vi "OperateControlPosition.vi"   [LabVIEW 2011]
uses:
  <vilib>/Utility/miscctls.llb/LVPositionTypeDef.ctl
types:
  T1 = typedef "LVPositionTypeDef.ctl" = cluster{"Left":i32, "Top":i32}
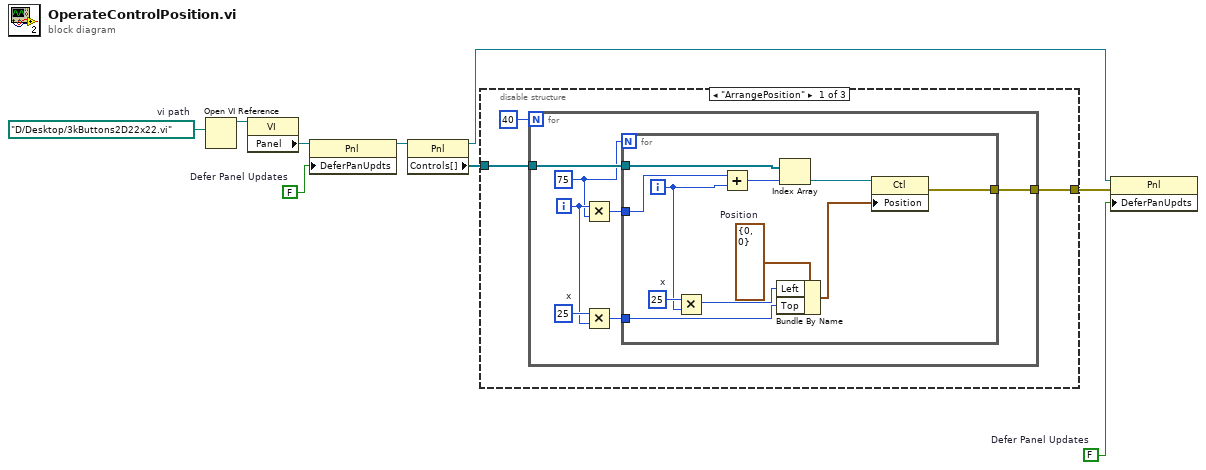
[diagram p0: block diagram]
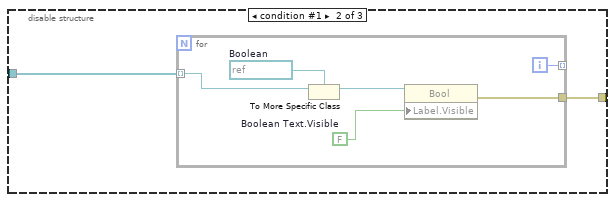
[diagram p2: hidden frame]
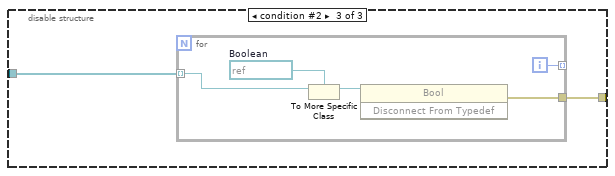
[diagram p3: hidden frame]
diagram:
  w3 = FALSE  # Defer Panel Updates
  w5 = FALSE  # Defer Panel Updates
  w7 = path "D:/Desktop/3kButtons2D22x22.vi"  # vi path
  n1 = Open VI Reference(vi path=w7) -> (vi reference=w8:refnum<vi>)  [unwired: 5 in, 1 out]
  n2 = property class="VI"(reference=w8) -> ("Panel"=w6:refnum<vi>)  [unwired: 1 in, 2 out]
  n3 = property class="Pnl"(reference=w6, "DeferPanUpdts"=w5) -> (reference out=w1:refnum<vi>)  [unwired: 1 in, 1 out]
  n4 = property class="Pnl"(reference=w1) -> (reference out=w2:refnum<vi>, "Controls[]"=w9:refnum<vi>[])  [unwired: 1 in, 1 out]
  n5 = disable-structure shown="\"ArrangePosition\"" {
    disable-tunnel: w9 -> [w12 w32 w40]
    disable-tunnel: [w11 w31 w39] -> w4
    frame condition #0 (active) {
      n6 = for {
        N: 40 -> [_]
        tunnel: w12 -> [w19]
        tunnel: [w18] -> w11
        i -> [w15]
        w17 = 25  # x
        w13 = 75
        n7 = Multiply(x=w15, y=w13) -> (x*y=w14:i32)
        n8 = Multiply(x=w17, y=w15) -> (x*y=w16:i32)
        n9 = for {
          N: w13 -> [_]
          tunnel: w19 -> [w30]
          tunnel: [w29] -> w18
          tunnel: w16 -> [w24]
          tunnel: w14 -> [w21]
          i -> [w20]
          w26 = 25  # x
          w28 = T1 {"Left"=0, "Top"=0}  # Position
          n10 = Multiply(x=w26, y=w20) -> (x*y=w25:i32)
          n11 = Add(x=w21, y=w20) -> (x+y=w22:i32)
          n12 = Bundle By Name(cluster=w28, "Left"=w25, "Top"=w24) -> (w27:T1)
          n13 = Index Array(array=w30, index=w22) -> (element=w23:refnum<vi>)
          n14 = property class="Ctl"(reference=w23, "Position"=w27) -> (error out=w29:errorcluster)  [unwired: 1 in, 1 out]
        }
      }
    }
    frame condition #1 {
      n15 = for {
        tunnel: w32 -> [w37] mode=indexing
        tunnel: [w38] -> w31
        tunnel: [w34] -> _ mode=indexing
        i -> [w34]
        w33 = FALSE  # Boolean Text.Visible
        w35 = refnum<vi> refnum  # Boolean
        n16 = To More Specific Class(target class=w35, reference=w37) -> (specific class reference=w36:refnum<vi>)  [unwired: 1 in, 1 out]
        n17 = property class="Bool"(reference=w36, "Label.Visible"=w33) -> (error out=w38:errorcluster)  [unwired: 1 in, 1 out]
      }
    }
    frame condition #2 {
      n18 = for {
        tunnel: w40 -> [w45] mode=indexing
        tunnel: [w43] -> _ mode=indexing
        tunnel: [w41] -> w39
        i -> [w43]
        w44 = refnum<vi> refnum  # Boolean
        n19 = To More Specific Class(target class=w44, reference=w45) -> (specific class reference=w42:refnum<vi>)  [unwired: 1 in, 1 out]
        n20 = invoke class="Bool" method="Disconnect From Typedef"(reference=w42) -> (error out=w41:errorcluster)  [unwired: 2 in, 2 out]
      }
    }
  }
  n21 = property class="Pnl"(reference=w2, error in=w4, "DeferPanUpdts"=w3) -> ()  [unwired: 2 out]
